vi "CXT info.vi"(8 "error in (no error)":errorcluster, 11 "Variant":variant) -> (0 "error out":errorcluster, 3 "child strings":string[](array[string]))   [LabVIEW 2017, in "Variant Tree API.lvlib"]
uses:
  Variant Tree/Source/Variant Tree API.lvlib
  <vilib>/Utility/Data Type/Get Numeric Information.vi
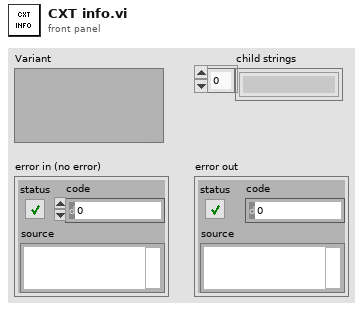
[diagram p1: front panel]
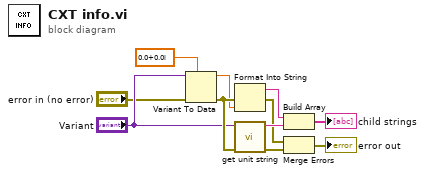
[diagram p0: block diagram]
diagram:
  n1 = Variant To Data(error in="error in (no error)", type=cdb 0.0+0.0i, Variant="Variant") -> (data=w2:cdb, error out=w9:errorcluster)
  n2 = Format Into String(error in=w9, w2) -> (resulting string=w3:string, error out=w6:errorcluster)  [unwired: 2 in]
  n3 = call "get unit string.vi"("error in (no error)"=w9, "Variant"="Variant") -> ("error out"=w11:errorcluster, "String"=w8:string)  [unwired: 8 in]
  n4 = Build Array(w3, w8) -> (→"child strings":string[])
  n5 = Merge Errors(w6, w11) -> (→"error out":errorcluster)
